vi "remove tag from table.vi"(9 "index":i32, 10 "data type":T1, 11 "data table in":T2) -> (3 "data table out":T2)   [LabVIEW 2013, in "tag bus.lvlib" / "data table.lvlib"]
doc: "Removes a specified tag, by type and index, from the data table."
uses:
  data table.lvlib
  data table.ctl
  tag/Data Type.ctl
  tag/tag descriptor.lvclass
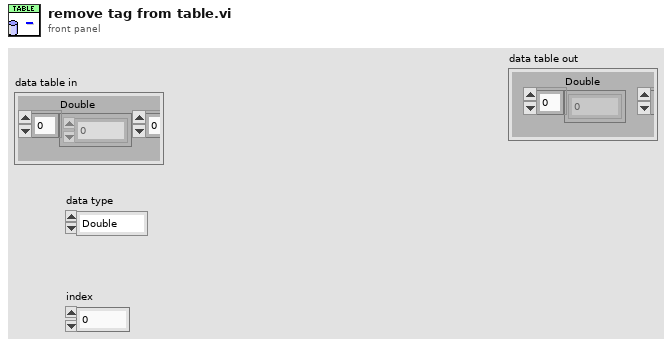
[diagram p1: front panel]
types:
  T1 = typedef "tag bus.lvlib/tag descriptor.lvclass/Data Type.ctl" = enum16{"Double", "Single", "I64", "I32", "I16", "I8", "U64", "U32", "U16", "U8", "Boolean", "String", "Array of Double", "Array of Single", "Array of I64", "Array of I32", "Array of I16", "Array of I8", "Array of U64", "Array of U32", "Array of U16", "Array of U8", "Array of Boolean", "Array of String"}
  T2 = typedef "tag bus.lvlib/data table.lvlib/data table.ctl" = cluster{"Double":dbl[], "Single":sgl[], "I64":i64[], "I32":i32[], "I16":i16[], "I8":i8[], "U64":u64[], "U32":u32[], "U16":u16[], "U8":u8[], "Boolean":bool[], "String":string[], "Array of Double":cluster{"DBL Array":dbl[]}[], "Array of Single":cluster{"SGL Array":sgl[]}[], "Array of I64":cluster{"I64 Array":i64[]}[], "Array of I32":cluster{"I32 Array":i32[]}[], "Array of I16":cluster{"I16 Array":i16[]}[], "Array of I8":cluster{"I8 Array":i8[]}[], "Array of U64":cluster{"U64 Array":u64[]}[], "Array of U32":cluster{"U32 Array":u32[]}[], "Array of U16":cluster{"U16 Array":u16[]}[], "Array of U8":cluster{"U8 Array":u8[]}[], "Array of Boolean":cluster{"Boolean Array":bool[]}[], "Array of String":cluster{"String Array":string[]}[]}
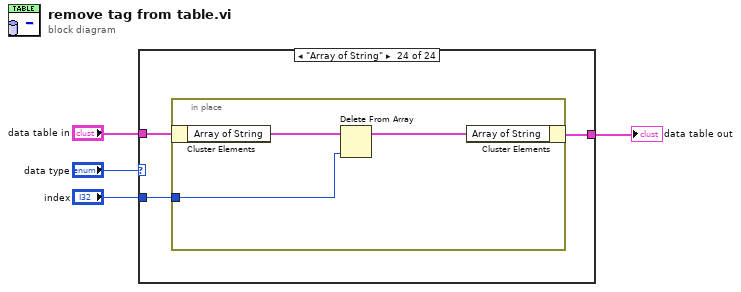
[diagram p0: block diagram]
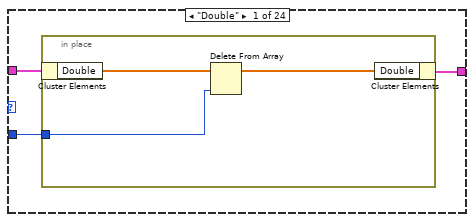
[diagram p2: hidden frame]
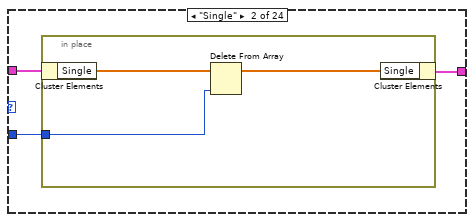
[diagram p3: hidden frame]
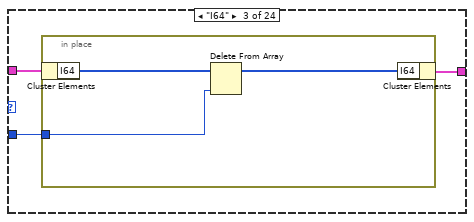
[diagram p4: hidden frame]
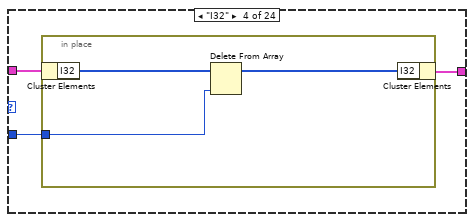
[diagram p5: hidden frame]
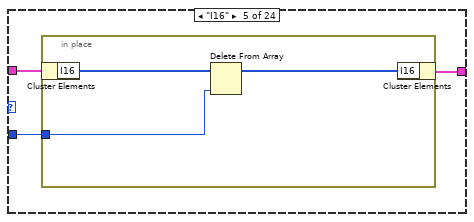
[diagram p6: hidden frame]
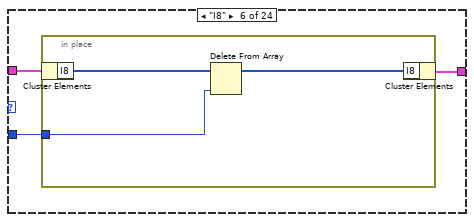
[diagram p7: hidden frame]
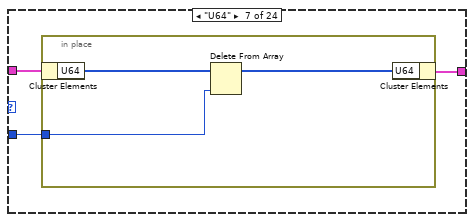
[diagram p8: hidden frame]
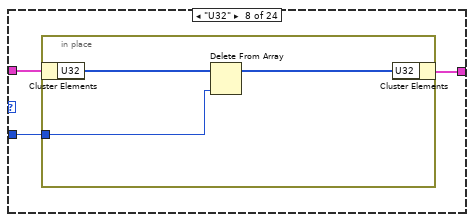
[diagram p9: hidden frame]
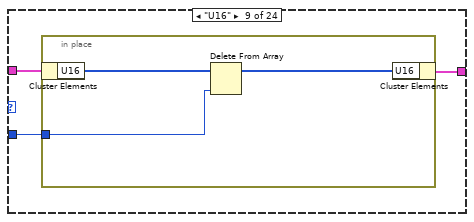
[diagram p10: hidden frame]
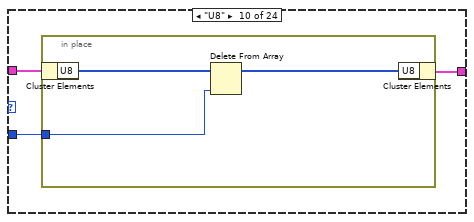
[diagram p11: hidden frame]
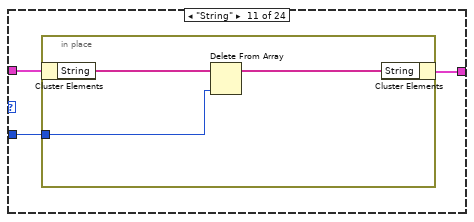
[diagram p12: hidden frame]
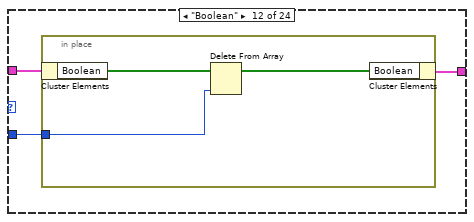
[diagram p13: hidden frame]
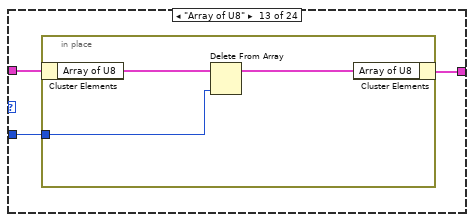
[diagram p14: hidden frame]
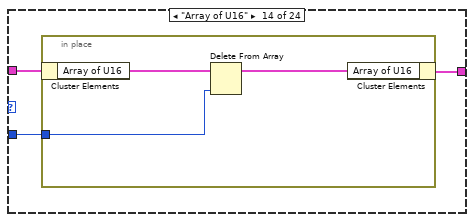
[diagram p15: hidden frame]
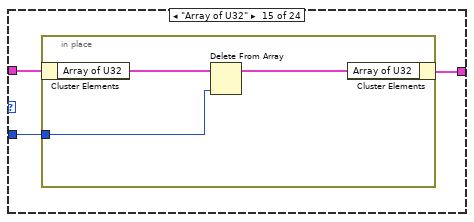
[diagram p16: hidden frame]
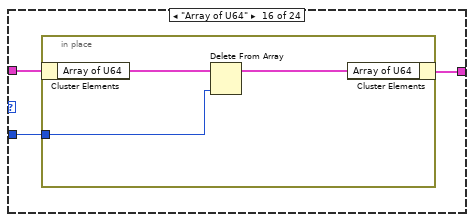
[diagram p17: hidden frame]
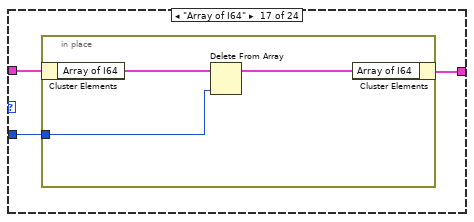
[diagram p18: hidden frame]
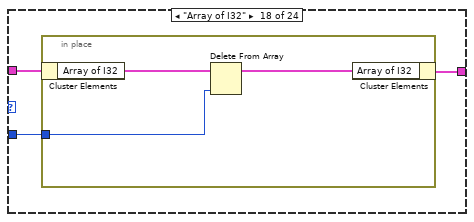
[diagram p19: hidden frame]
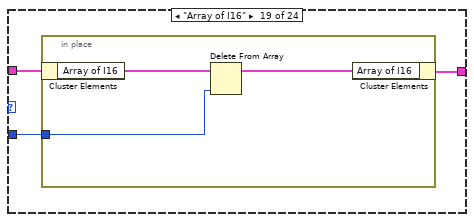
[diagram p20: hidden frame]
diagram:
  n1 = case shown="\"Array of String\"" "data type" {
    tunnel: "data table in" -> [w7 w13 w19 w25 w31 w37 w43 w49 w55 w61 w67 w73 w79 w85 w91 w97 w103 w109 w115 w121 w127 w133 w139 w145]
    tunnel: [w6 w12 w18 w24 w30 w36 w42 w48 w54 w60 w66 w72 w78 w84 w90 w96 w102 w108 w114 w120 w126 w132 w138 w144] -> w3
    tunnel: "index" -> [w5 w11 w17 w23 w29 w35 w41 w47 w53 w59 w65 w71 w77 w83 w89 w95 w101 w107 w113 w119 w125 w131 w137 w143]
    frame "Double" {
      n2 = in-place {
        in-place-border: w5 -> [w8]
        n3 = in-place-cluster #1(w7) -> ("Double"=w10:dbl[])
        n4 = Delete From Array(array=w10, index=w8) -> (array with subset deleted=w9:dbl[])  [unwired: 1 in, 1 out]
        n5 = in-place-cluster #1("Double"=w9) -> (w6:T2)
      }
    }
    frame "Single" {
      n6 = in-place {
        in-place-border: w11 -> [w14]
        n7 = in-place-cluster #2(w13) -> ("Single"=w16:sgl[])
        n8 = Delete From Array(array=w16, index=w14) -> (array with subset deleted=w15:sgl[])  [unwired: 1 in, 1 out]
        n9 = in-place-cluster #2("Single"=w15) -> (w12:T2)
      }
    }
    frame "I64" {
      n10 = in-place {
        in-place-border: w17 -> [w20]
        n11 = in-place-cluster #3(w19) -> ("I64"=w22:i64[])
        n12 = Delete From Array(array=w22, index=w20) -> (array with subset deleted=w21:i64[])  [unwired: 1 in, 1 out]
        n13 = in-place-cluster #3("I64"=w21) -> (w18:T2)
      }
    }
    frame "I32" {
      n14 = in-place {
        in-place-border: w23 -> [w26]
        n15 = in-place-cluster #4(w25) -> ("I32"=w28:i32[])
        n16 = Delete From Array(array=w28, index=w26) -> (array with subset deleted=w27:i32[])  [unwired: 1 in, 1 out]
        n17 = in-place-cluster #4("I32"=w27) -> (w24:T2)
      }
    }
    frame "I16" {
      n18 = in-place {
        in-place-border: w29 -> [w32]
        n19 = in-place-cluster #5(w31) -> ("I16"=w34:i16[])
        n20 = Delete From Array(array=w34, index=w32) -> (array with subset deleted=w33:i16[])  [unwired: 1 in, 1 out]
        n21 = in-place-cluster #5("I16"=w33) -> (w30:T2)
      }
    }
    frame "I8" {
      n22 = in-place {
        in-place-border: w35 -> [w38]
        n23 = in-place-cluster #6(w37) -> ("I8"=w40:i8[])
        n24 = Delete From Array(array=w40, index=w38) -> (array with subset deleted=w39:i8[])  [unwired: 1 in, 1 out]
        n25 = in-place-cluster #6("I8"=w39) -> (w36:T2)
      }
    }
    frame "U64" {
      n26 = in-place {
        in-place-border: w41 -> [w44]
        n27 = in-place-cluster #7(w43) -> ("U64"=w46:u64[])
        n28 = Delete From Array(array=w46, index=w44) -> (array with subset deleted=w45:u64[])  [unwired: 1 in, 1 out]
        n29 = in-place-cluster #7("U64"=w45) -> (w42:T2)
      }
    }
    frame "U32" {
      n30 = in-place {
        in-place-border: w47 -> [w50]
        n31 = in-place-cluster #8(w49) -> ("U32"=w52:u32[])
        n32 = Delete From Array(array=w52, index=w50) -> (array with subset deleted=w51:u32[])  [unwired: 1 in, 1 out]
        n33 = in-place-cluster #8("U32"=w51) -> (w48:T2)
      }
    }
    frame "U16" {
      n34 = in-place {
        in-place-border: w53 -> [w56]
        n35 = in-place-cluster #9(w55) -> ("U16"=w58:u16[])
        n36 = Delete From Array(array=w58, index=w56) -> (array with subset deleted=w57:u16[])  [unwired: 1 in, 1 out]
        n37 = in-place-cluster #9("U16"=w57) -> (w54:T2)
      }
    }
    frame "U8" {
      n38 = in-place {
        in-place-border: w59 -> [w62]
        n39 = in-place-cluster #10(w61) -> ("U8"=w64:u8[])
        n40 = Delete From Array(array=w64, index=w62) -> (array with subset deleted=w63:u8[])  [unwired: 1 in, 1 out]
        n41 = in-place-cluster #10("U8"=w63) -> (w60:T2)
      }
    }
    frame "String" {
      n42 = in-place {
        in-place-border: w65 -> [w68]
        n43 = in-place-cluster #11(w67) -> ("String"=w70:string[])
        n44 = Delete From Array(array=w70, index=w68) -> (array with subset deleted=w69:string[])  [unwired: 1 in, 1 out]
        n45 = in-place-cluster #11("String"=w69) -> (w66:T2)
      }
    }
    frame "Boolean" {
      n46 = in-place {
        in-place-border: w71 -> [w74]
        n47 = in-place-cluster #12(w73) -> ("Boolean"=w76:bool[])
        n48 = Delete From Array(array=w76, index=w74) -> (array with subset deleted=w75:bool[])  [unwired: 1 in, 1 out]
        n49 = in-place-cluster #12("Boolean"=w75) -> (w72:T2)
      }
    }
    frame "Array of U8" {
      n50 = in-place {
        in-place-border: w77 -> [w80]
        n51 = in-place-cluster #13(w79) -> ("Array of U8"=w82:cluster{"U8 Array":u8[]}[])
        n52 = Delete From Array(array=w82, index=w80) -> (array with subset deleted=w81:cluster{"U8 Array":u8[]}[])  [unwired: 1 in, 1 out]
        n53 = in-place-cluster #13("Array of U8"=w81) -> (w78:T2)
      }
    }
    frame "Array of U16" {
      n54 = in-place {
        in-place-border: w83 -> [w86]
        n55 = in-place-cluster #14(w85) -> ("Array of U16"=w88:cluster{"U16 Array":u16[]}[])
        n56 = Delete From Array(array=w88, index=w86) -> (array with subset deleted=w87:cluster{"U16 Array":u16[]}[])  [unwired: 1 in, 1 out]
        n57 = in-place-cluster #14("Array of U16"=w87) -> (w84:T2)
      }
    }
    frame "Array of U32" {
      n58 = in-place {
        in-place-border: w89 -> [w92]
        n59 = in-place-cluster #15(w91) -> ("Array of U32"=w94:cluster{"U32 Array":u32[]}[])
        n60 = Delete From Array(array=w94, index=w92) -> (array with subset deleted=w93:cluster{"U32 Array":u32[]}[])  [unwired: 1 in, 1 out]
        n61 = in-place-cluster #15("Array of U32"=w93) -> (w90:T2)
      }
    }
    frame "Array of U64" {
      n62 = in-place {
        in-place-border: w95 -> [w98]
        n63 = in-place-cluster #16(w97) -> ("Array of U64"=w100:cluster{"U64 Array":u64[]}[])
        n64 = Delete From Array(array=w100, index=w98) -> (array with subset deleted=w99:cluster{"U64 Array":u64[]}[])  [unwired: 1 in, 1 out]
        n65 = in-place-cluster #16("Array of U64"=w99) -> (w96:T2)
      }
    }
    frame "Array of I64" {
      n66 = in-place {
        in-place-border: w101 -> [w104]
        n67 = in-place-cluster #17(w103) -> ("Array of I64"=w106:cluster{"I64 Array":i64[]}[])
        n68 = Delete From Array(array=w106, index=w104) -> (array with subset deleted=w105:cluster{"I64 Array":i64[]}[])  [unwired: 1 in, 1 out]
        n69 = in-place-cluster #17("Array of I64"=w105) -> (w102:T2)
      }
    }
    frame "Array of I32" {
      n70 = in-place {
        in-place-border: w107 -> [w110]
        n71 = in-place-cluster #18(w109) -> ("Array of I32"=w112:cluster{"I32 Array":i32[]}[])
        n72 = Delete From Array(array=w112, index=w110) -> (array with subset deleted=w111:cluster{"I32 Array":i32[]}[])  [unwired: 1 in, 1 out]
        n73 = in-place-cluster #18("Array of I32"=w111) -> (w108:T2)
      }
    }
    frame "Array of I16" {
      n74 = in-place {
        in-place-border: w113 -> [w116]
        n75 = in-place-cluster #19(w115) -> ("Array of I16"=w118:cluster{"I16 Array":i16[]}[])
        n76 = Delete From Array(array=w118, index=w116) -> (array with subset deleted=w117:cluster{"I16 Array":i16[]}[])  [unwired: 1 in, 1 out]
        n77 = in-place-cluster #19("Array of I16"=w117) -> (w114:T2)
      }
    }
    frame "Array of I8" {
      n78 = in-place {
        in-place-border: w119 -> [w122]
        n79 = in-place-cluster #20(w121) -> ("Array of I8"=w124:cluster{"I8 Array":i8[]}[])
        n80 = Delete From Array(array=w124, index=w122) -> (array with subset deleted=w123:cluster{"I8 Array":i8[]}[])  [unwired: 1 in, 1 out]
        n81 = in-place-cluster #20("Array of I8"=w123) -> (w120:T2)
      }
    }
    frame "Array of Double" {
      n82 = in-place {
        in-place-border: w125 -> [w128]
        n83 = in-place-cluster #21(w127) -> ("Array of Double"=w130:cluster{"DBL Array":dbl[]}[])
        n84 = Delete From Array(array=w130, index=w128) -> (array with subset deleted=w129:cluster{"DBL Array":dbl[]}[])  [unwired: 1 in, 1 out]
        n85 = in-place-cluster #21("Array of Double"=w129) -> (w126:T2)
      }
    }
    frame "Array of Single" {
      n86 = in-place {
        in-place-border: w131 -> [w134]
        n87 = in-place-cluster #22(w133) -> ("Array of Single"=w136:cluster{"SGL Array":sgl[]}[])
        n88 = Delete From Array(array=w136, index=w134) -> (array with subset deleted=w135:cluster{"SGL Array":sgl[]}[])  [unwired: 1 in, 1 out]
        n89 = in-place-cluster #22("Array of Single"=w135) -> (w132:T2)
      }
    }
    frame "Array of Boolean" {
      n90 = in-place {
        in-place-border: w137 -> [w140]
        n91 = in-place-cluster #23(w139) -> ("Array of Boolean"=w142:cluster{"Boolean Array":bool[]}[])
        n92 = Delete From Array(array=w142, index=w140) -> (array with subset deleted=w141:cluster{"Boolean Array":bool[]}[])  [unwired: 1 in, 1 out]
        n93 = in-place-cluster #23("Array of Boolean"=w141) -> (w138:T2)
      }
    }
    frame "Array of String" {
      n94 = in-place {
        in-place-border: w143 -> [w146]
        n95 = in-place-cluster #24(w145) -> ("Array of String"=w148:cluster{"String Array":string[]}[])
        n96 = Delete From Array(array=w148, index=w146) -> (array with subset deleted=w147:cluster{"String Array":string[]}[])  [unwired: 1 in, 1 out]
        n97 = in-place-cluster #24("Array of String"=w147) -> (w144:T2)
      }
    }
  }
  "data table out" <- w3
